vi "Reset credit.vi"(8 "error in (no error)":errorcluster, 10 "Compra realizada":bool, 11 "MXN Actor in":refnum<class "MXN Actor.lvclass">) -> (0 "error out":errorcluster, 3 "MXN Actor out":refnum<class "MXN Actor.lvclass">)   [LabVIEW 2020, in "MXN Actor.lvlib" / "MXN Actor.lvclass"]
uses:
  MXN Actor.lvclass
  MXN Actor.lvclass/MXN Actor.ctl
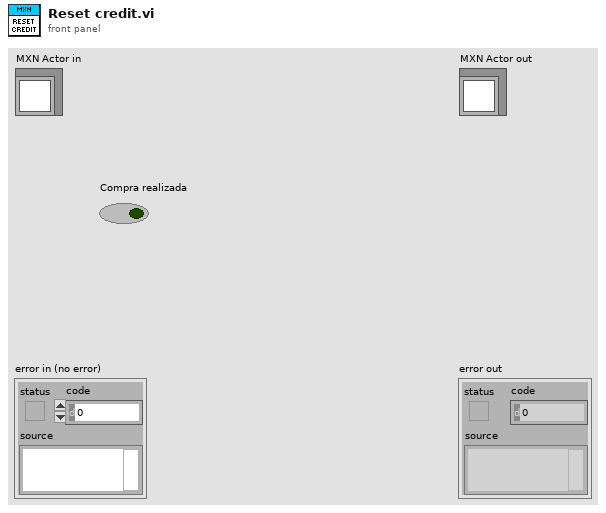
[diagram p1: front panel]
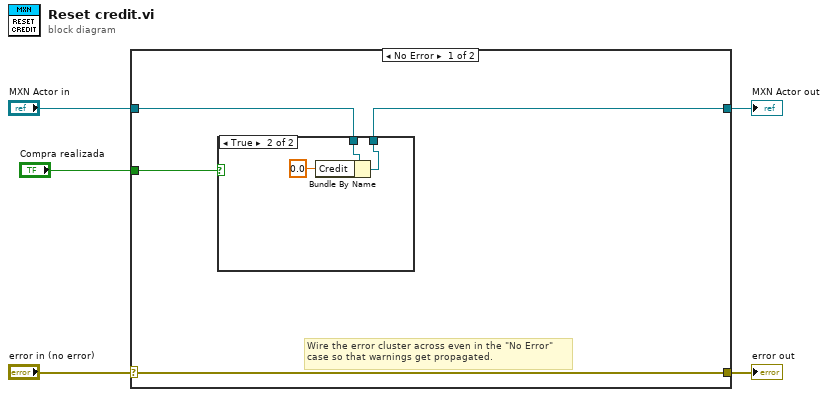
[diagram p0: block diagram]
diagram:
  n1 = case shown="No Error" "error in (no error)" {
    selector: "error in (no error)" -> [w9 w15]
    tunnel: [w9 w15] -> w4
    tunnel: [w6 w14] -> w2
    tunnel: "MXN Actor in" -> [w7 w14]
    tunnel: "Compra realizada" -> [w8 _]
    frame No Error {
      # "Wire the error cluster across even in the \"No Error\"\ncase so that warnings get propagated."
      n2 = case shown="True" w8 {
        tunnel: w7 -> [w10 w13]
        tunnel: [w10 w12] -> w6
        frame False {
        }
        frame True {
          n3 = Bundle By Name(cluster=w13, "Credit"=0.0) -> (w12:refnum<class "MXN Actor.lvclass">)
        }
      }
    }
    frame Error {
    }
  }
  "error out" <- w4
  "MXN Actor out" <- w2
